vi "Test 1D Fit.vi"() -> ()   [LabVIEW 2021, in "Fits.lvlib"]
uses:
  Fit Models.ctl
  Power Law/Power Law Fit Parameters.ctl
  Fit Settings.ctl
  Nonlinear Fit Method.ctl
  Ramp Type.ctl
  Residual Type.ctl
  Non-linear Fitting Algorithm.ctl
  My Fit Stopping Criteria.ctl
  Graphs/XY Graph/XY Graph Refnum.ctl
  1D Fit Simulation Options.ctl
  Fit Plot Request Information.ctl
  <vilib>/Utility/miscctls.llb/LVPointDoubleTypeDef.ctl
  Fits.lvlib
  Graphs/XY Graph/XY Graph Add-Ons.lvlib
panel:
  in  "Tab Control":enum32{"Data & Fit", "Options"}(tab)
  out "Fit ouput":string
  out "Graph":cluster{"X Array":dbl[], "Y Array":dbl[]}[](graph)
  out "Graph TipStrip":string
  in  "# Points":i32=100
  in  "Fit Models":T1
  in  "X min":dbl
  in  "X max":dbl
  in  "Noise?":bool
  in  "Noise Model":enum16{"Gaussian", "Poisson"}(ring)
  in  "Gaussian Noise SDV":dbl
  in  "Simulate":bool
  in  "Fit":bool
  in  "Power Law Fit Parameters":T2
  in  "Fit Settings":T3={"Use Original Plot # Points"=TRUE, "# Fit Plot Points"=0, "Fitting Method"=enum."Least Square", "Weighted Fit"=TRUE, "Show All Fit Components"=FALSE, "Axis Type"=0, "Show Fit Residuals"=TRUE, "Residual Type"=enum."Standard", "Fitting Algorithm"=enum."Levenberg-Marquardt"} {"Axis Type" items=["Linear", "Logarithmic"]}
  in  "Termination Criteria":T8={"Max Iterations"=1000, "Max Function Calls"=10000, "Max Time"=1000.0, "Function Tolerance"=1e-06, "Parameter Tolerance"=1e-06, "Gradient Tolerance"=1e-06, "Min Lambda"=1e-06, "Max Lambda"=1000000.0, "Initial Tick Count"=0}
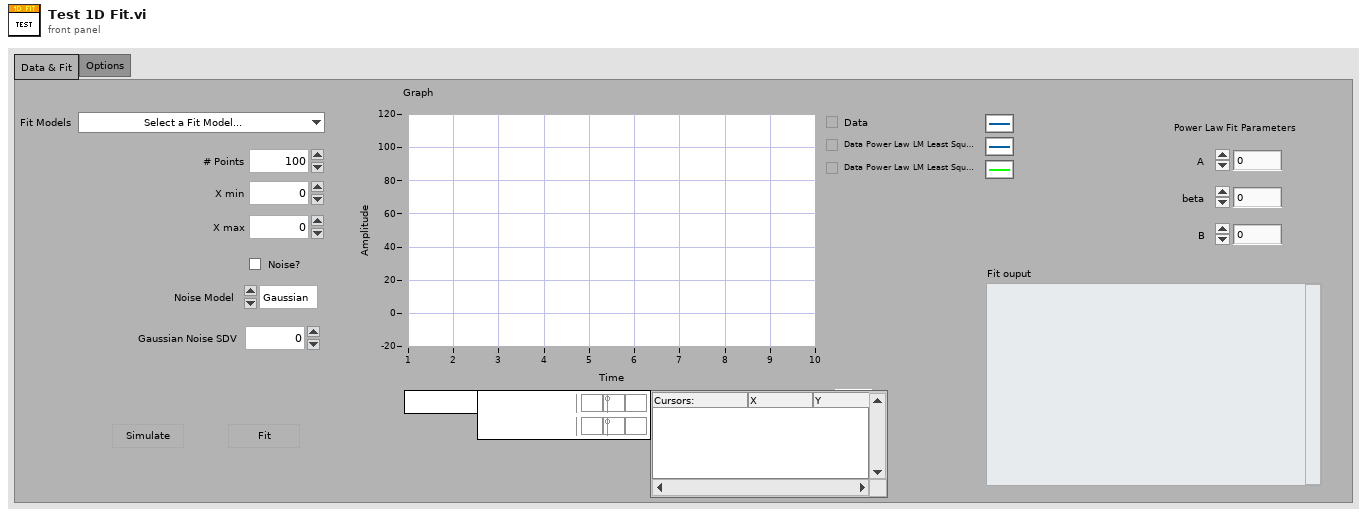
[diagram p1: front panel]
types:
  T1 = typedef "Fits.lvlib/Fit Models.ctl" = enum16{"Select a Fit Model...", "           Single Peak", "Gaussian", "Asymmetric Gaussian", "Lorentzian", "Asymmetric Lorentzian", "Gaussian/Lorentzian", "Lorentzian/Gaussian", "           Double Peak", "Two Gaussians", "Two Asymmetric Gaussians", "Two H-Connected Gaussians", "Two T-Connected Gaussians", "Two H-Connected Asymmetric Gaussians", "Two T-Connected Asymmetric Gaussians", "           Triple Peak", "Three Gaussians", "Three Asymmetric Gaussians", "              Decays", "1-Exponential", "IRF*PSED", "2-Exponentials", "Power Law", "               ACF", "2D Gaussian ACF", "2D Gaussian + Blinking ACF", "2D Gaussian + Flow ACF", "3D Gaussian ACF", "3D Gaussian + Blinking ACF", "             Multiplot", "2D Gaussian ACF & 2D Gaussian + Flow ACF"}
  T2 = typedef "Fits.lvlib/Power Law Fit Parameters.ctl" = cluster{"A":dbl, "beta":dbl, "B":dbl, "Mean":dbl, "SDV":dbl, "Integral":dbl, "MSE":dbl, "R^2":dbl}
  T3 = typedef "Fits.lvlib/Fit Settings.ctl" = cluster{"Use Original Plot # Points":bool, "# Fit Plot Points":u32, "Fitting Method":T4, "Weighted Fit":bool, "Show All Fit Components":bool, "Axis Type":T5, "Show Fit Residuals":bool, "Residual Type":T6, "Fitting Algorithm":T7}
  T4 = typedef "Fits.lvlib/Nonlinear Fit Method.ctl" = enum16{"Least Square", "Least Absolute Residual", "Bisquare", "MLE"}
  T5 = typedef "Fits.lvlib/Ramp Type.ctl" = u16
  T6 = typedef "Fits.lvlib/Residual Type.ctl" = enum16{"Standard", "Normalized", "Reduced"}
  T7 = typedef "Fits.lvlib/Non-linear Fitting Algorithm.ctl" = enum16{"Levenberg-Marquardt", "Trust-Region Dogleg"}
  T8 = typedef "Fits.lvlib/My Fit Stopping Criteria.ctl" = cluster{"Max Iterations":i32, "Max Function Calls":i32, "Max Time":dbl[unit], "Function Tolerance":dbl, "Parameter Tolerance":dbl, "Gradient Tolerance":dbl, "Min Lambda":dbl, "Max Lambda":dbl, "Initial Tick Count":u32}
  T9 = cluster{"XY Graph TipStrip":refnum<event-registration>}
  T10 = typedef "Fits.lvlib/1D Fit Simulation Options.ctl" = cluster{"Fit Models":T1, "# Points":i32, "X max":dbl, "X min":dbl, "Noise?":bool, "Noise Model":enum16{"Gaussian", "Poisson"}, "Gaussian Noise SDV":dbl}
  T11 = typedef "Fits.lvlib/Fit Plot Request Information.ctl" = cluster{"XY Graph Ref":refnum<vi>, "Mouse Coordinates":T12, "Fit Model":T1, "Plot Index":i32}
  T12 = typedef "LVPointDoubleTypeDef.ctl" = cluster{"X":dbl, "Y":dbl}
  T13 = typedef "LVPoint32TypeDef.ctl" = cluster{"Horizontal":i32, "Vertical":i32}
  T14 = typedef "XY Graph Add-Ons.lvlib/XY Plot Data.ctl" = cluster{"X Array":dbl[], "Y Array":dbl[]}
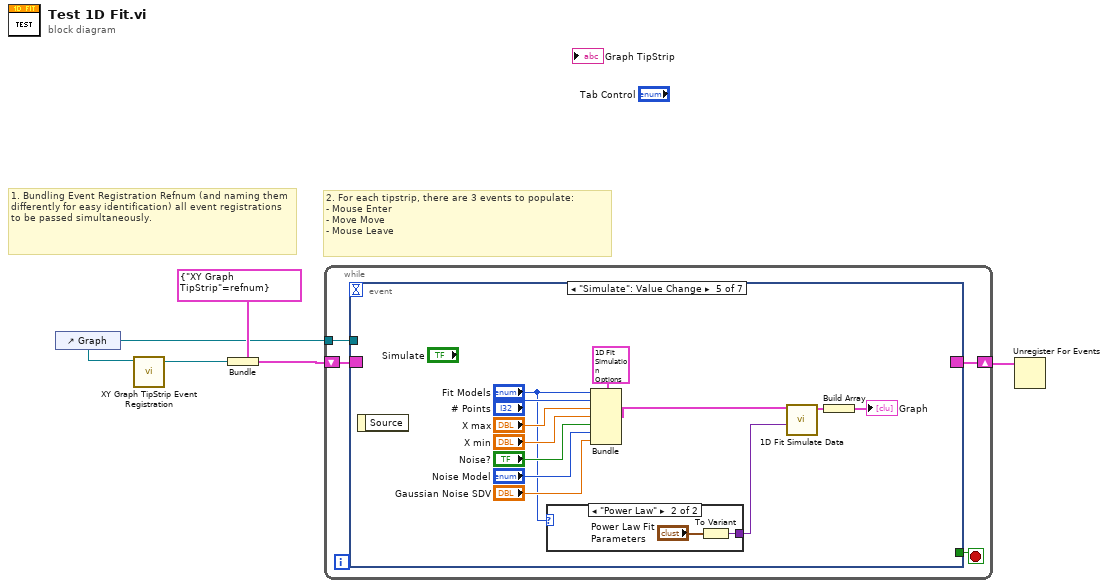
[diagram p0: block diagram]
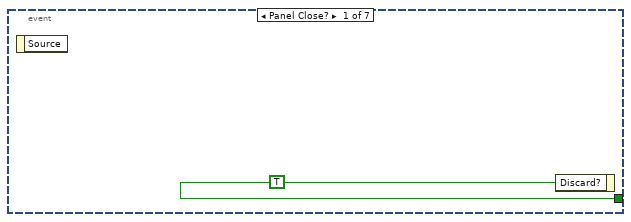
[diagram p2: hidden frame]
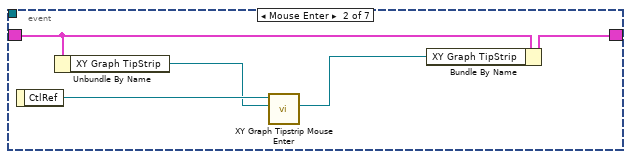
[diagram p3: hidden frame]
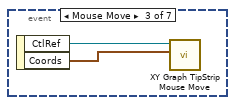
[diagram p4: hidden frame]
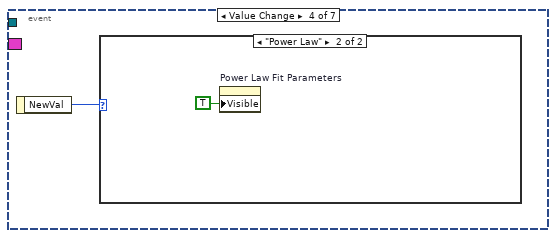
[diagram p5: hidden frame]
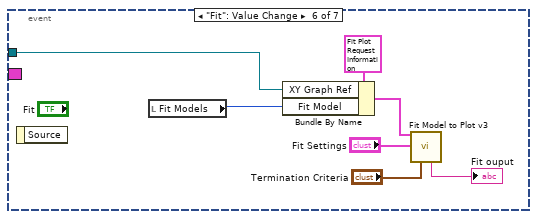
[diagram p8: hidden frame]
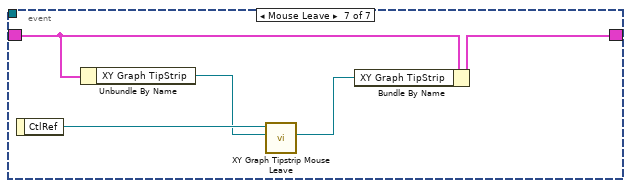
[diagram p9: hidden frame]
diagram:
  # "2. For each tipstrip, there are 3 events to populate:\n- Mouse Enter\n- Move Move\n- Mouse Leave"
  # "1. Bundling Event Registration Refnum (and naming them differently for easy identification) all event registrations to be passed simultaneously."
  n1 = control-ref of="Graph"() -> (w1:refnum<vi>)
  n2 = call "XY Graph TipStrip Event Registration.vi"("XY Graph Refnum"=w1) -> ("Event Registration Refnum"=w2:refnum<event-registration>)  [unwired: 8 in, 2 out]
  n3 = Bundle(cluster=T9 {"XY Graph TipStrip"=refnum} ("Event Registration Refnums"), "XY Graph TipStrip"=w2) -> (w4:T9)
  n4 = while {
    shift-right: [w7] -> w3
    shift-left: w4 -> [w9]
    tunnel: w1 -> [w6]
    stop <- w8 stop-if-true
    n5 = event shown="[4] \"Simulate\": Value Change" {
      selector: w9 -> [_ w13 _ _ _ _ w42]
      dyn-events: [_ w15 _ _ _ _ w41] -> w7
      timeout: _ -> [_ _ _ _ _ _ _]
      tunnel: [w10 _ _ _ _ _ _] -> w8
      tunnel: w6 -> [_ _ _ _ _ w34 _]
      event Panel Close? {
        w10 = TRUE ("Discard?")
        n6 = event-data() -> ()  [unwired: 1 in, 1 out]
        n7 = event-data("Discard?"=w10) -> ()  [unwired: 1 in, 1 out]
      }
      event Mouse Enter {
        n8 = event-data() -> ("CtlRef"=w14:refnum<vi>)  [unwired: 1 in]
        n9 = Unbundle By Name(w13) -> ("XY Graph TipStrip"=w12:refnum<event-registration>)
        n10 = call "XY Graph Tipstrip Mouse Enter.vi"("Event Registration Refnum"=w12, "XY Graph Refnum"=w14) -> ("Event Registration Refnum"=w11:refnum<event-registration>)  [unwired: 8 in, 1 out]
        n11 = Bundle By Name(cluster=w13, "XY Graph TipStrip"=w11) -> (w15:T9)
      }
      event Mouse Move {
        n12 = event-data() -> ("CtlRef"=w17:refnum<vi>, "Coords"=w16:T13)  [unwired: 1 in]
        n13 = call "XY Graph TipStrip Mouse Move.vi"("Coords"=w16, "XY Graph Refnum"=w17) -> ()  [unwired: 7 in, 3 out]
      }
      event Value Change {
        n14 = event-data() -> ("NewVal"=w18:T1)  [unwired: 1 in]
        n15 = case shown="\"Power Law\"" w18 {
          frame "Select a Fit Model...", Default {
          }
          frame "Power Law" {
            n16 = property on="Power Law Fit Parameters" class="Clust (strict)"("Visible"=TRUE) -> ()  [unwired: 2 in, 2 out]
          }
        }
      }
      event "Simulate": Value Change {
        n17 = event-data() -> ()  [unwired: 1 in, 1 out]
        n18 = case shown="\"Power Law\"" "Fit Models" {
          tunnel: [_ w32] -> w22
          frame "Select a Fit Model...", Default {
          }
          frame "Power Law" {
            n19 = To Variant(anything="Power Law Fit Parameters") -> (Variant=w32:variant)
          }
        }
        n20 = Bundle(cluster=T10 {"Fit Models"=enum."Select a Fit Model...", "# Points"=0, "X max"=0.0, "X min"=0.0, "Noise?"=FALSE, "Noise Model"=enum."Gaussian", "Gaussian Noise SDV"=0.0}, "Fit Models"="Fit Models", "# Points"="# Points", "X max"="X max", "X min"="X min", "Noise?"="Noise?", "Noise Model"="Noise Model", "Gaussian Noise SDV"="Gaussian Noise SDV") -> (w23:T10)
        n21 = call "1D Fit Simulate Data.vi"("Model Parameters"=w22, "Simulation Options"=w23) -> ("Plot"=w20:T14)  [unwired: 8 in, 1 out]
        n22 = Build Array(w20) -> (→"Graph":T14[])
      }
      event "Fit": Value Change {
        n23 = event-data() -> ()  [unwired: 1 in, 1 out]
        n24 = local read "Fit Models"() -> (w35:T1)
        n25 = Bundle By Name(cluster=T11 {"XY Graph Ref"=refnum, "Mouse Coordinates"={"X"=nan, "Y"=nan}, "Fit Model"=enum."Select a Fit Model...", "Plot Index"=0} ("Fit Plot Information"), "XY Graph Ref"=w34, "Fit Model"=w35) -> (w37:T11)
        n26 = call "Fit Model to Plot v3.vi"("Fit Plot Information"=w37, "Fit Settings"="Fit Settings", "Termination Criteria"="Termination Criteria") -> ("Fit Result String"=→"Fit ouput":string)  [unwired: 4 in, 8 out]
      }
      event Mouse Leave {
        n27 = event-data() -> ("CtlRef"=w45:refnum<vi>)  [unwired: 1 in]
        n28 = Unbundle By Name(w42) -> ("XY Graph TipStrip"=w44:refnum<event-registration>)
        n29 = call "XY Graph Tipstrip Mouse Leave.vi"("Event Registration Refnum"=w44, "XY Graph Refnum"=w45) -> ("Event Registration Refnum"=w43:refnum<event-registration>)  [unwired: 8 in, 1 out]
        n30 = Bundle By Name(cluster=w42, "XY Graph TipStrip"=w43) -> (w41:T9)
      }
    }
  }
  n31 = Unregister For Events(event registration refnum=w3) -> ()  [unwired: 1 in, 1 out]
